vi "Delete Aux Diagram.vi"(11 "tsRef":refnum<vi>) -> (3 "tsRef out":refnum<vi>)   [LabVIEW 2020, in "NI_TargetHelper.lvlib"]
uses:
  <vilib>/TargetSupport/NI_TargetHelper/NI_TargetHelper.lvlib
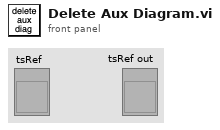
[diagram p1: front panel]
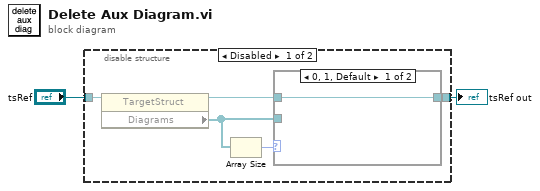
[diagram p0: block diagram]
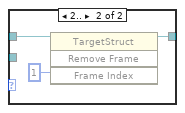
[diagram p2: hidden frame]
diagram:
  n1 = disable-structure shown="Disabled" {
    disable-tunnel: "tsRef" -> [w7 w12]
    disable-tunnel: [w3 w12] -> w1
    frame Disabled {
      n2 = property class="TargetStruct"(reference=w7) -> (reference out=w4:refnum<vi>, "Diagrams"=w5:refnum<vi>[])  [unwired: 1 in, 1 out]
      n3 = Array Size(array=w5) -> (size(s)=w6:i32)
      n4 = case shown="0, 1, Default" w6 {
        tunnel: w5 -> [_ _]
        tunnel: w4 -> [w8 w11]
        tunnel: [w8 w9] -> w3
        frame 0, 1, Default {
        }
        frame 2.. {
          n5 = invoke class="TargetStruct" method="Remove Frame"(reference=w11, "Frame Index"=u32 1) -> (reference out=w9:refnum<vi>)  [unwired: 2 in, 3 out]
        }
      }
    }
    frame Enabled {
    }
  }
  "tsRef out" <- w1
